vi "Write Set DER SetPointV Msg.vi"(10 "Set DER SetPointV Msg":refnum<class "Set DER SetPointV Msg.lvclass">, 11 "SCADA Sub Abstract in":refnum<class "Device Communication and Control Abstract.lvclass">) -> (3 "SCADA Sub Abstract out":refnum<class "Device Communication and Control Abstract.lvclass">)   [LabVIEW 2018, in "Device Communication and Control Abstract Actor.lvlib" / "Device Communication and Control Abstract.lvclass"]
uses:
  Device Communication and Control Abstract.lvclass
  Device Communication and Control Abstract Messages/Set DER SetPointV Msg/Set DER SetPointV Msg.lvclass
  Device Communication and Control Abstract.lvclass/Device Communication and Control Abstract.ctl
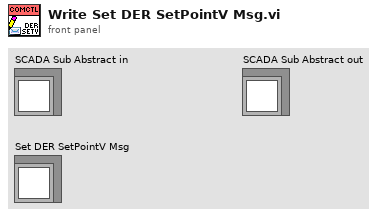
[diagram p1: front panel]
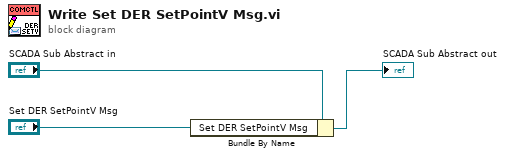
[diagram p0: block diagram]
diagram:
  n1 = Bundle By Name(cluster="SCADA Sub Abstract in", "Set DER SetPointV Msg"="Set DER SetPointV Msg") -> (→"SCADA Sub Abstract out":refnum<class "Device Communication and Control Abstract.lvclass">)
